vi "Extract Field.vi"(11 "Buffer in":u8[](array[numeric]) format="%.0x") -> (2 "Field Data":u8[](array[numeric])=[0, 0, 0, 0, 0, 0, 240, 63, 0, 0, 0, 0, 0, 0, 0, 64, 0, 0, 0, 0, 0, 0, 8, 64, 0, 0, 0, 0, 0, 0, 16, 64] format="%.0x", 3 "Buffer":u8[](array[numeric]) format="%.0x", 5 "Wire Type":T1, 7 "Field Number":i32)   [LabVIEW 2020, in "LV-Proto.lvlib"]
uses:
  LV-Proto.lvlib
  Wire Type.ctl
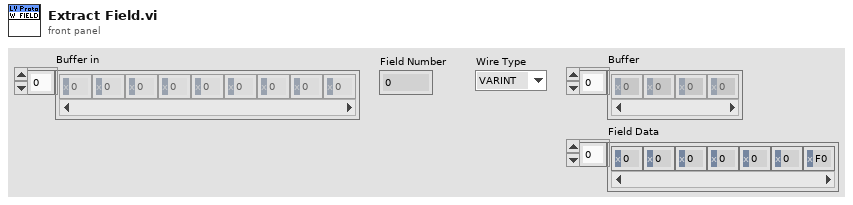
[diagram p1: front panel]
types:
  T1 = typedef "LV-Proto.lvlib/Wire Type.ctl" = enum8{"VARINT", "I64", "LEN", "SGROUP (Deprecated)", "EGROUP (Deprecated)", "I32"}
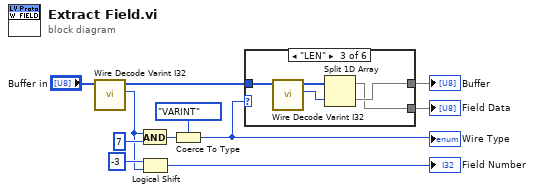
[diagram p0: block diagram]
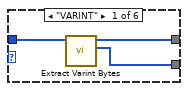
[diagram p2: hidden frame]
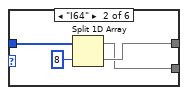
[diagram p3: hidden frame]
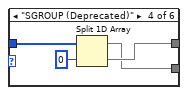
[diagram p4: hidden frame]
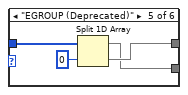
[diagram p5: hidden frame]
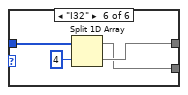
[diagram p6: hidden frame]
diagram:
  n1 = call "Wire Decode Varint I32.vi"("Buffer in"="Buffer in") -> ("I32"=w8:i32, "Buffer"=w3:u8[])  [unwired: 9 in]
  n2 = And(x=w8, y=7) -> (x .and. y?=w6:i32)
  n3 = Logical Shift(y=i16 -3, x=w8) -> (x << y=→"Field Number":i32)
  n4 = Coerce To Type(0:w6, 1:Wire_Type."VARINT" ("Wire Type")) -> (2:w4:T1)
  "Wire Type" <- w4
  n5 = case shown="\"LEN\"" w4 {
    tunnel: w3 -> [w14 w18 w23 w27 w31 w35]
    tunnel: [w13 w16 w20 w25 w29 w33] -> w2
    tunnel: [w12 w15 w19 w24 w28 w32] -> w1
    frame "VARINT" {
      n6 = call "Extract Varint Bytes.vi"("Buffer in"=w14) -> ("Varint Bytes"=w12:u8[], "Buffer"=w13:u8[])  [unwired: 9 in]
    }
    frame "I64" {
      n7 = Split 1D Array(array=w18, index=8) -> (first subarray=w15:u8[], second subarray=w16:u8[])
    }
    frame "LEN" {
      n8 = call "Wire Decode Varint I32.vi"("Buffer in"=w23) -> ("I32"=w21:i32, "Buffer"=w22:u8[])  [unwired: 9 in]
      n9 = Split 1D Array(array=w22, index=w21) -> (first subarray=w19:u8[], second subarray=w20:u8[])
    }
    frame "SGROUP (Deprecated)" {
      n10 = Split 1D Array(array=w27, index=0) -> (first subarray=w24:u8[], second subarray=w25:u8[])
    }
    frame "EGROUP (Deprecated)" {
      n11 = Split 1D Array(array=w31, index=0) -> (first subarray=w28:u8[], second subarray=w29:u8[])
    }
    frame "I32" {
      n12 = Split 1D Array(array=w35, index=4) -> (first subarray=w32:u8[], second subarray=w33:u8[])
    }
  }
  "Buffer" <- w2
  "Field Data" <- w1
